vi "Read Communication.vi"(8 "error in (no error)":errorcluster, 11 "SiemensDigitalEnergyMeter in":refnum<class "SiemensDigitalEnergyMeter.lvclass">) -> (0 "error out":errorcluster, 2 "Communication":T1, 3 "SiemensDigitalEnergyMeter out":refnum<class "SiemensDigitalEnergyMeter.lvclass">)   [LabVIEW 2018, in "SensorPlugins.lvlib" / "SiemensDigitalEnergyMeter.lvclass"]
uses:
  SiemensDigitalEnergyMeter.lvclass
  TypeDefinitions/CommunicationControls.ctl
  <vilib>/NI/Modbus Library/API/Master/Modbus Master.lvclass
  SiemensDigitalEnergyMeter.lvclass/SiemensDigitalEnergyMeter.ctl
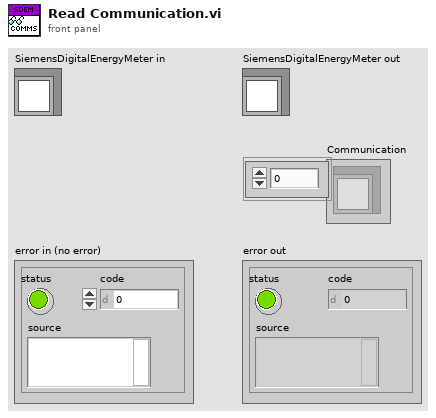
[diagram p1: front panel]
types:
  T1 = typedef "SensorPlugins.lvlib/SiemensDigitalEnergyMeter.lvclass/CommunicationControls.ctl" = refnum<class "Modbus Master.lvclass">[]
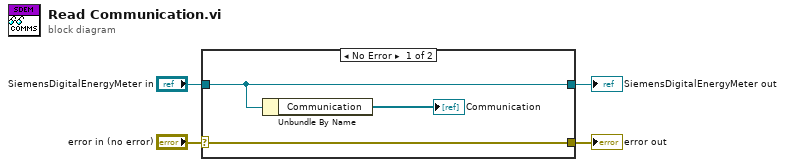
[diagram p0: block diagram]
diagram:
  n1 = case shown="No Error" "error in (no error)" {
    selector: "error in (no error)" -> [w7 w9]
    tunnel: [w7 w9] -> w3
    tunnel: [w6 w8] -> w1
    tunnel: "SiemensDigitalEnergyMeter in" -> [w6 w8]
    frame No Error {
      n2 = Unbundle By Name(w6) -> ("Communication"=→"Communication":T1)
    }
    frame Error {
    }
  }
  "error out" <- w3
  "SiemensDigitalEnergyMeter out" <- w1
